vi "init_spectrometers.vi"(1 "spectrIdx":u16, 5 "error in (no error)":errorcluster) -> (14 "nr spectr found":i32, 19 "error out":errorcluster)   [LabVIEW 2010, in "OSA.lvclass"]
doc: "Lower level init routine, higher level routines will be sufficient in most cases."
uses:
  OSA.lvclass
  FTSLib.dll
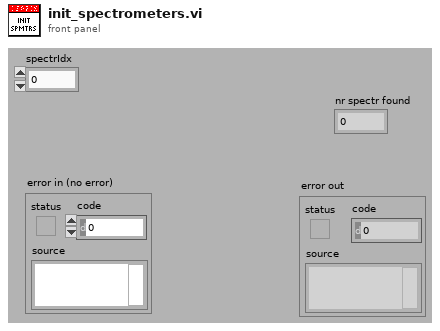
[diagram p1: front panel]
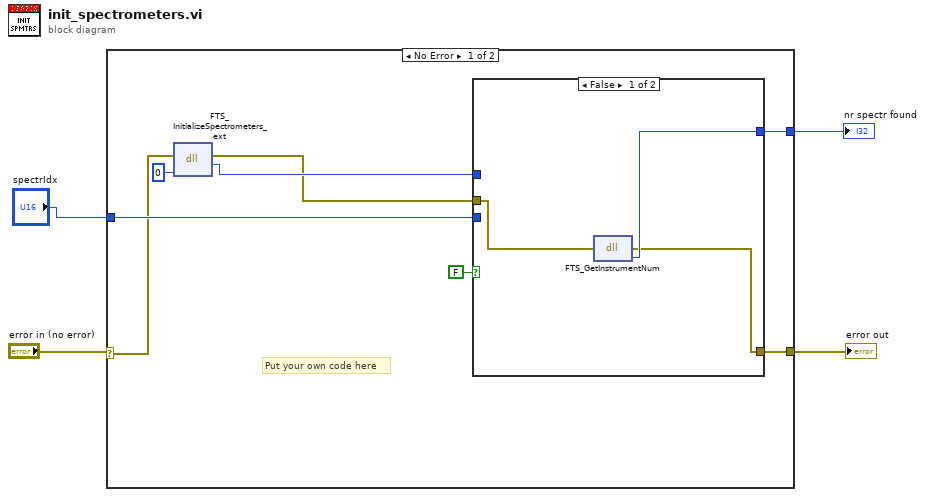
[diagram p0: block diagram]
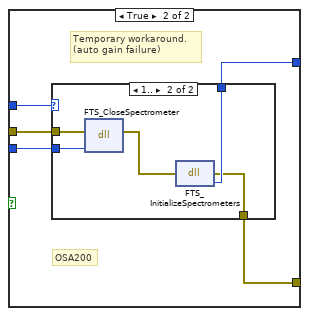
[diagram p2: hidden frame]
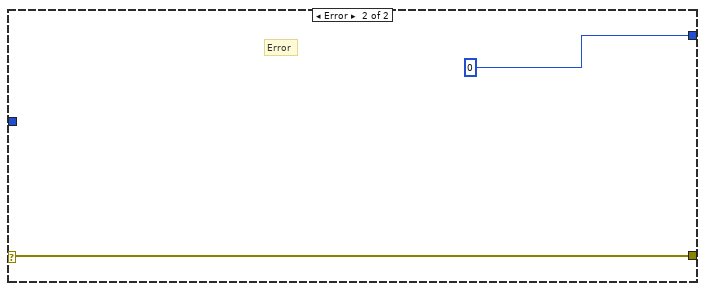
[diagram p4: hidden frame]
diagram:
  n1 = case shown="No Error" "error in (no error)" {
    selector: "error in (no error)" -> [w8 w29]
    tunnel: [w11 w29] -> w4
    tunnel: [w12 0] -> w2
    tunnel: "spectrIdx" -> [w10 _]
    frame No Error {
      # "Put your own code here"
      n2 = dll-call lib="FTSLib.dll" fn="FTS_InitializeSpectrometers_ext"(error in=w8, "nullPtr"=u64 0) -> (error out=w7:errorcluster, "return type"=w9:i32)  [unwired: 3 in, 1 out]
      n3 = case shown="False" FALSE {
        tunnel: [w15 w20] -> w12
        tunnel: [w13 w19] -> w11
        tunnel: w10 -> [_ w18]
        tunnel: w9 -> [_ w17]
        tunnel: w7 -> [w14 w16]
        frame False {
          n4 = dll-call lib="FTSLib.dll" fn="FTS_GetInstrumentNum"(error in=w14) -> (error out=w13:errorcluster, "return type"=w15:i32)  [unwired: 2 in, 1 out]
        }
        frame True {
          # "OSA200"
          # "Temporary workaround.\n(auto gain failure)"
          n5 = case shown="1.." w17 {
            selector: w17 -> [w22 _]
            tunnel: [w22 w27] -> w20
            tunnel: [w21 w26] -> w19
            tunnel: w18 -> [_ w24]
            tunnel: w16 -> [w21 w23]
            frame 0, Default {
            }
            frame 1.. {
              n6 = dll-call lib="FTSLib.dll" fn="FTS_CloseSpectrometer"(error in=w23, "spectrIdx"=w24) -> (error out=w25:errorcluster)  [unwired: 4 in, 1 out]
              n7 = dll-call lib="FTSLib.dll" fn="FTS_InitializeSpectrometers"(error in=w25) -> (error out=w26:errorcluster, "return type"=w27:i32)  [unwired: 2 in, 1 out]
            }
          }
        }
      }
    }
    frame Error {
      # "Error"
    }
  }
  "error out" <- w4
  "nr spectr found" <- w2
